vi "Amplitude and Levels.vi"   [LabVIEW 2020, in "NI_MAPro.lvlib"]
doc: "Returns the <B>amplitude</B>, <B>high state level</B>, and <B>low state level</B> of a waveform or an array of waveforms. Wire data to the <B>signal in</B> input to determine the polymorphic instance to use or manually select the instance."
uses:
  NI_MAPro.lvlib
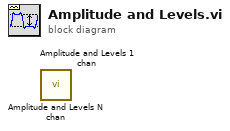
[diagram p0: block diagram]
diagram:
  n1 = call "Amplitude and Levels N chan.vi"() -> ()  [unwired: 8 in, 4 out]
  n2 = call "Amplitude and Levels 1 chan.vi"() -> ()  [unwired: 8 in, 4 out]
